vi "Set_Control_Values_by_Index_(Sgnl).vi"(7 "Control References":refnum<vi>[](array[refnum]), 8 "error in (no error)":errorcluster, 9 "appended array":variant[](array[variant]), 11 "VI Refnum":refnum<vi>) -> (0 "error out":errorcluster, 3 "VI Refnum":refnum<vi>)   [LabVIEW 2015]
panel:
  out "appended array 2":variant[](array[variant])
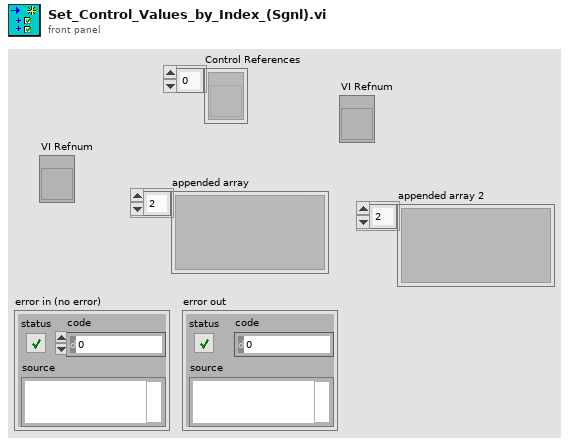
[diagram p1: front panel]
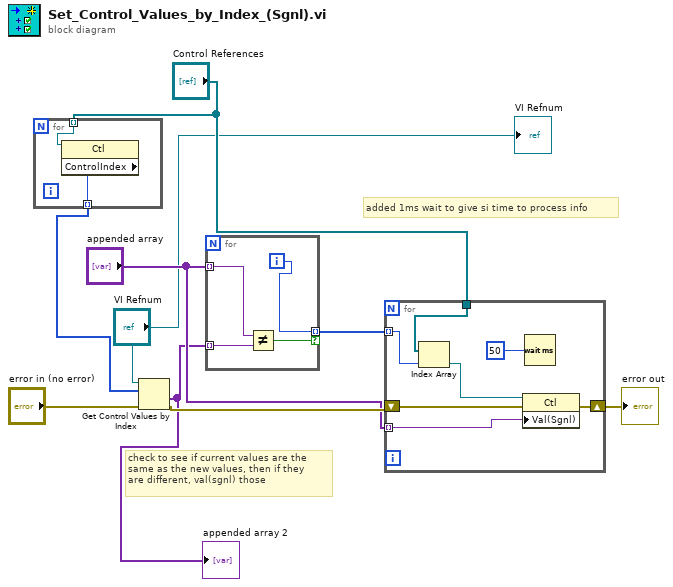
[diagram p0: block diagram]
diagram:
  # "check to see if current values are the \nsame as the new values, then if they\nare different, val(sgnl) those"
  # "added 1ms wait to give si time to process info"
  n1 = for {
    tunnel: "Control References" -> [w11] mode=indexing
    tunnel: [w10] -> w5 mode=indexing
    n2 = property class="Ctl"(reference=w11) -> ("ControlIndex"=w10:i32)  [unwired: 1 in, 2 out]
  }
  n3 = Get Control Values by Index(0:"VI Refnum", 1:w5, 3:"error in (no error)") -> (10:w1:variant[], 11:w4:errorcluster)
  "appended array 2" <- w1
  n4 = for {
    tunnel: "appended array" -> [w15] mode=indexing
    tunnel: w1 -> [w14] mode=indexing
    tunnel: [w12] -> w9 mode=indexing if=w13
    i -> [w12]
    n5 = Not Equal?(x=w15, y=w14) -> (x != y?=w13:bool)
  }
  n6 = for {
    tunnel: w9 -> [w20] mode=indexing
    shift-right: [w22] -> w7
    shift-left: w4 -> [w17]
    tunnel: "Control References" -> [w21]
    tunnel: "appended array" -> [w16] mode=indexing
    n7 = Index Array(array=w21, index=w20) -> (element=w18:refnum<vi>)
    n8 = property class="Ctl"(reference=w18, error in=w17, "Val(Sgnl)"=w16) -> (error out=w22:errorcluster)  [unwired: 1 out]
    n9 = Wait (ms)(milliseconds to wait=50) -> ()  [unwired: 1 out]
  }
  "error out" <- w7
  "VI Refnum" <- "VI Refnum"
